vi "Pointer.Throughput.vi"() -> ()   [LabVIEW 2016]
uses:
  <vilib>/Platform/TimedLoop/XDataNode/timing_clust.ctl
  <vilib>/Platform/TimedLoop/XDataNode/nitl_modes.ctl
  <vilib>/Platform/TimedLoop/XDataNode/wakeup.ctl
  Library/Classes/Pointer/Memory.Pointer.lvclass/Memory.Pointer.ctl
  Library/Classes/Pointer/Methods/Memory.Pointer.Allocate.vi
  Library/Classes/Pointer/Methods/Accessors/Memory.Pointer.Get Address.vi
  Library/Classes/Pointer/Methods/Memory.Pointer.Offset to Address.Unsafe.vi
  Library/VIs/Memory.Move.vi
  Library/Classes/Pointer/Methods/Accessors/Memory.Pointer.Set Address.vi
  Library/Classes/Pointer/Methods/Accessors/Memory.Pointer.Set Size.vi
  Library/Classes/Pointer/Methods/Memory.Pointer.Parameter Check.Size.vi
  Library/VIs/Memory.Truncate I64 to I32.vi
  <vilib>/platform/TimedLoop/XDataNode/XDataNode.xnode
  Library/Classes/Pointer/Memory.Pointer.lvclass
  <vilib>/Platform/TimedLoop/XDataNode/XDNodeRunTimeDep.lvlib
panel:
  in  "start size":i64=1000 format="%.0pB"
  in  "number of transfers":i32=1000
  in  "end size":i64=1000000 format="%.0pB"
  out "Throughput":cluster{"X":dbl, "Y":dbl}[](graph)
  out "Peak Throughput":dbl format="%.3pB/s"
  in  "iterations":i32=100
  in  "processor":i32=-2
  out "allocated size":i64=2147483647 format="%d bytes"
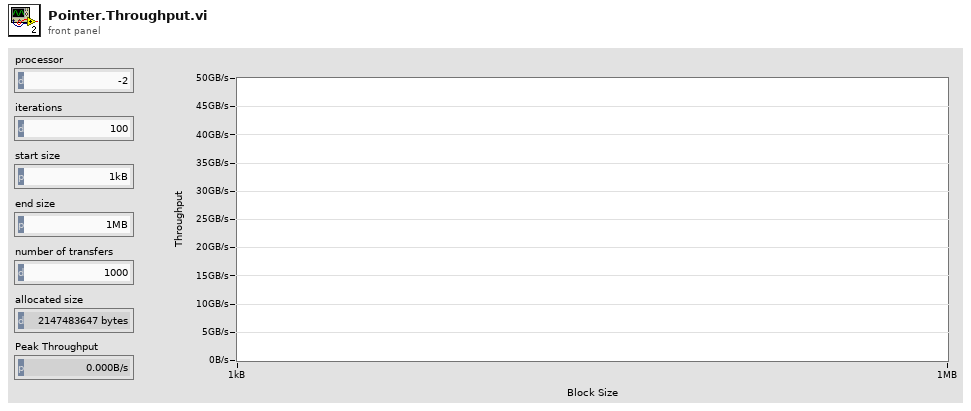
[diagram p1: front panel]
types:
  T1 = typedef "XDNodeRunTimeDep.lvlib/timing_clust.ctl" = cluster{"Expected End [f-1]":u64, "Actual End [f-1]":u64, "Finished Late? [f-1]":bool, "Expected End [i-1]":u64, "Actual End [i-1]":u64, "Finished Late? [i-1]":bool, "Expected Start [i]":u64, "Actual Start [i]":u64, "Expected Start [f]":u64, "Actual Start [f]":u64, "Source Name":string, "Structure Name":string, "Period":i64, "Deadline":i64, "Offset":i64, "Start":i64, "Priority":i32, "Timeout":i32, "Mode":T2, "Wakeup Reason":T3, "Error":errorcluster, "Source Type":string, "Secondary Source Type":string, "Global End Time":u64, "Global Start Time":u64, "Frame Duration":u64, "Iteration Duration":u64, "Assigned CPU":i32, "I/O Scan Engine Mode":u32}
  T2 = typedef "XDNodeRunTimeDep.lvlib/nitl_modes.ctl" = enum32{"No Change", "Process missed periods, maintain original phase", "Discard missed periods, maintain original phase", "Process missed periods, ignore original phase", "Discard missed periods, ignore original phase"}
  T3 = typedef "XDNodeRunTimeDep.lvlib/wakeup.ctl" = enum32{"Normal", "Aborted", "Asynchronous wakeup", "Timing source error", "Timed loop error", "Timeout"}
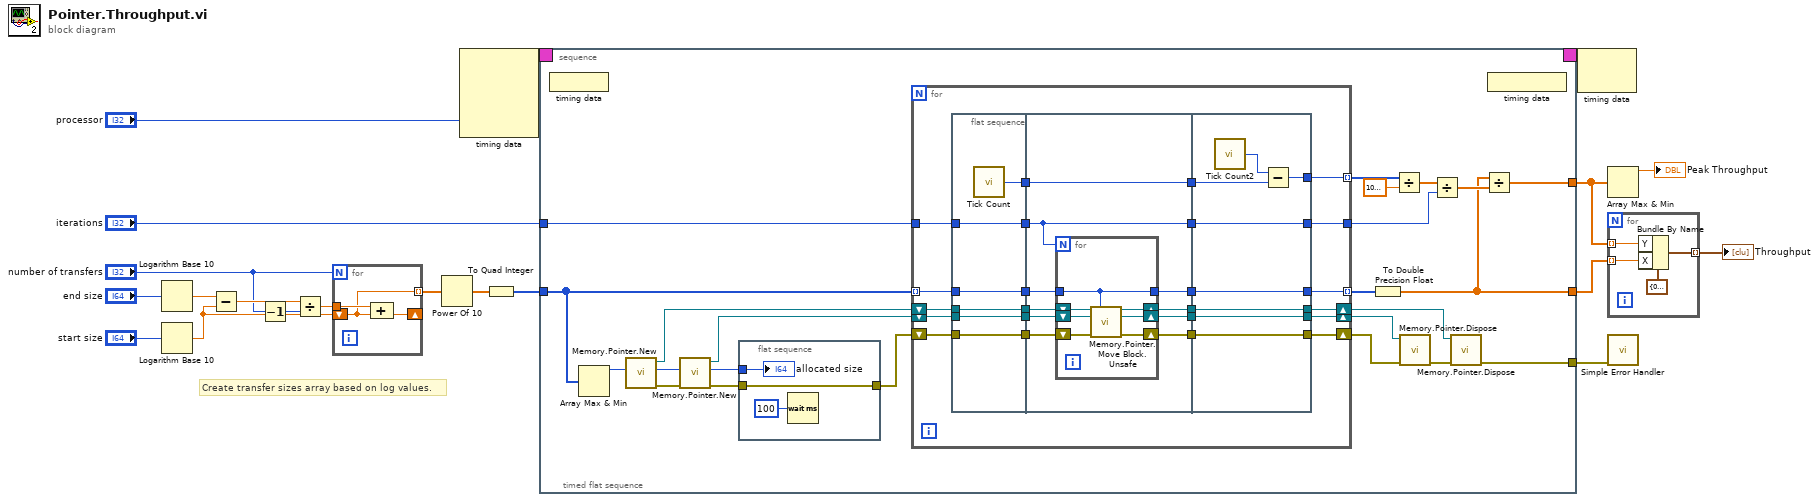
[diagram p0: block diagram]
diagram:
  # "Create transfer sizes array based on log values."
  n1 = Logarithm Base 10(1:"end size") -> (0:w9:dbl)
  n2 = Logarithm Base 10(1:"start size") -> (0:w6:dbl)
  n3 = Subtract(x=w9, y=w6) -> (x-y=w8:dbl)
  n4 = Decrement(x="number of transfers") -> (x-1=w4:i32)
  n5 = Divide(x=w8, y=w4) -> (x/y=w7:dbl)
  n6 = for {
    N: "number of transfers" -> [_]
    tunnel: w7 -> [w23]
    shift-right: [w22] -> _
    shift-left: w6 -> [w21]
    tunnel: [w21] -> w3 mode=indexing
    n7 = Compound Arithmetic op=ADD(w23, w21) -> (w22:dbl)
  }
  n8 = Power Of 10(x=w3) -> (10^x=w2:dbl[])
  n9 = node-c288("processor") -> (w20:T1)  [unwired: 3 in]
  n10 = To Quad Integer(1:w2) -> (0:w1:i64[])
  n11 = timed-sequence {
    timing: w20 -> [_]
    timing-out: [_] -> w19
    tunnel: "iterations" -> [w28]
    tunnel: [w27] -> w16
    tunnel: [w26] -> w14
    tunnel: w1 -> [w25]
    tunnel: [w24] -> w13
    n12 = timed-flat-sequence {
      tunnel: w28 -> [w29]
      tunnel: [w44] -> w27
      tunnel: [w42] -> w26
      tunnel: w25 -> [w40]
      tunnel: [w30] -> w24
      n13 = node-c288() -> ()  [unwired: 1 in]
      n14 = Array Max & Min(array=w40) -> (max value=w39:i64)  [unwired: 3 out]
      n15 = call "Memory.Pointer.New.vi"("size"=w39) -> ("error out"=w49:errorcluster, "allocated size"=w35:i64, "Pointer out"=w50:refnum<class "Memory.Pointer.lvclass">)  [unwired: 8 in]
      n16 = call "Memory.Pointer.New.vi"("error in (no error)"=w49, "size"=w35) -> ("error out"=w34:errorcluster, "allocated size"=w36:i64, "Pointer out"=w51:refnum<class "Memory.Pointer.lvclass">)  [unwired: 7 in]
      n17 = flat-sequence {
        tunnel: w36 -> [w52]
        tunnel: w34 -> [w53]
        tunnel: [w53] -> w33
        frame #0 {
          n18 = Wait (ms)(milliseconds to wait=u32 100) -> ()  [unwired: 1 out]
          "allocated size" <- w52
        }
      }
      n19 = for {
        shift-right: [w62] -> w47
        shift-left: w51 -> [w66]
        shift-right: [w61] -> w45
        shift-left: w50 -> [w65]
        shift-right: [w63] -> w48
        shift-left: w33 -> [w64]
        tunnel: [w59] -> w38 mode=indexing
        tunnel: w40 -> [w58] mode=indexing
        tunnel: [w57] -> w31 mode=indexing
        tunnel: w29 -> [w67]
        tunnel: [w60] -> w43
        n20 = flat-sequence {
          tunnel: [w85] -> w79
          tunnel: [w84] -> w78
          tunnel: [w83] -> w77
          tunnel: [w82] -> w76
          tunnel: [w81] -> w75
          tunnel: [w80] -> w74
          tunnel: w65 -> [w85]
          tunnel: w66 -> [w84]
          tunnel: w64 -> [w83]
          tunnel: w58 -> [w82]
          tunnel: w67 -> [w81]
          tunnel: w79 -> [w95]
          tunnel: w78 -> [w94]
          tunnel: w77 -> [w93]
          tunnel: w76 -> [w92]
          tunnel: w75 -> [w88]
          tunnel: w74 -> [w87]
          tunnel: [w87] -> w73
          tunnel: [w91] -> w72
          tunnel: [w90] -> w71
          tunnel: [w89] -> w70
          tunnel: [w88] -> w69
          tunnel: [w86] -> w68
          tunnel: w73 -> [w109]
          tunnel: w72 -> [w108]
          tunnel: [w108] -> w63
          tunnel: w71 -> [w107]
          tunnel: w70 -> [w106]
          tunnel: [w107] -> w61
          tunnel: [w106] -> w62
          tunnel: w69 -> [w105]
          tunnel: [w105] -> w60
          tunnel: w68 -> [w104]
          tunnel: [w104] -> w57
          tunnel: [w103] -> w59
          frame #0 {
            n21 = call "Tick Count"() -> ("Tick Count(uSec)"=w80:u32)
          }
          frame #1 {
            n22 = for {
              N: w88 -> [_]
              shift-right: [w99] -> w91
              shift-left: w93 -> [w100]
              shift-right: [w98] -> w90
              shift-left: w95 -> [w102]
              shift-right: [w97] -> w89
              shift-left: w94 -> [w101]
              tunnel: w92 -> [w96]
              tunnel: [w96] -> w86
              n23 = call "Memory.Pointer.Move Block.Unsafe.vi"("src Pointer in"=w102, "length"=w96, "dst Pointer in"=w101, "error in (no error)"=w100) -> ("src Pointer out"=w98:refnum<class "Memory.Pointer.lvclass">, "dst Pointer out"=w97:refnum<class "Memory.Pointer.lvclass">, "error out"=w99:errorcluster)  [unwired: 9 in]
            }
          }
          frame #2 {
            n24 = call "Tick Count2"() -> ("Tick Count(uSec)"=w110:u32)
            n25 = Subtract(x=w110, y=w109) -> (x-y=w103:u32)
          }
        }
      }
      n26 = To Double Precision Float(number=w31) -> (double precision float=w30:dbl[])
      n27 = Divide(x=w38, y=1000000.0) -> (x/y=w37:dbl[])
      n28 = call "Memory.Pointer.Dispose.vi"("error in (no error)"=w48, "Pointer in"=w47) -> ("error out"=w46:errorcluster)  [unwired: 9 in]
      n29 = Divide(x=w37, y=w43) -> (x/y=w32:dbl[])
      n30 = call "Memory.Pointer.Dispose.vi"("error in (no error)"=w46, "Pointer in"=w45) -> ("error out"=w44:errorcluster)  [unwired: 9 in]
      n31 = Divide(x=w30, y=w32) -> (x/y=w42:dbl[])
      n32 = node-c288() -> ()  [unwired: 1 out]
    }
  }
  n33 = node-c288(w19) -> ()  [unwired: 1 out]
  n34 = Array Max & Min(array=w14) -> (max value=→"Peak Throughput":dbl)  [unwired: 3 out]
  n35 = for {
    tunnel: w14 -> [w112] mode=indexing
    tunnel: w13 -> [w113] mode=indexing
    tunnel: [w111] -> w12 mode=indexing
    n36 = Bundle By Name(cluster=cluster{"X":dbl, "Y":dbl} {"X"=0.0, "Y"=0.0}, "Y"=w112, "X"=w113) -> (w111:cluster{"X":dbl, "Y":dbl})
  }
  "Throughput" <- w12
  n37 = call <vilib>:"Simple Error Handler.vi"("error in (no error)"=w16) -> ()  [unwired: 4 in, 5 out]
